vi "VersionCompareIn4Num.vi"(11 "VersionOnWeb":string) -> (3 "realFoundNew":bool)   [LabVIEW 2015]
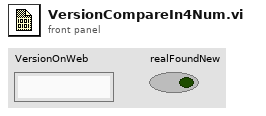
[diagram p1: front panel]
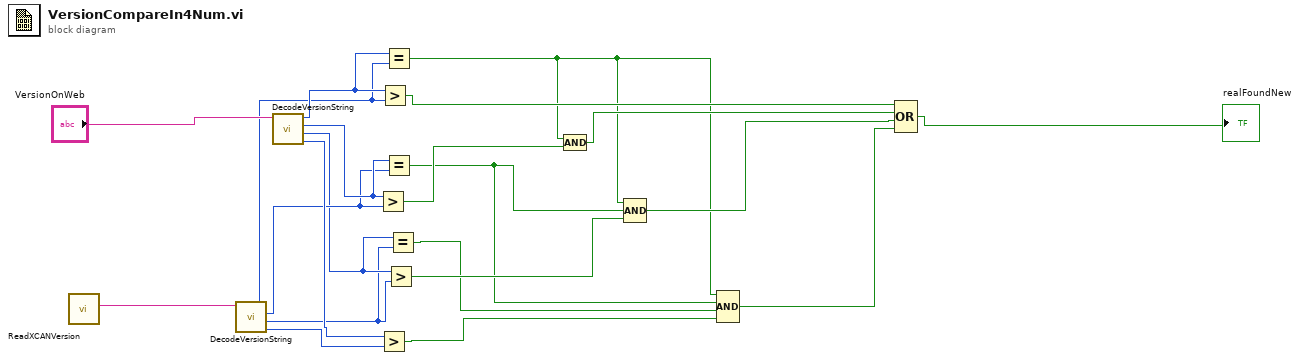
[diagram p0: block diagram]
diagram:
  n1 = call "ReadXCANVersion.vi"() -> ("Version"=w20:string)  [unwired: 9 in, 1 out]
  n2 = call "DecodeVersionString.vi"("VersionStr"=w20) -> ("build"=w18:i32, "correction"=w11:i32, "secondary"=w13:i32, "Main"=w15:i32)  [unwired: 5 in]
  n3 = call "DecodeVersionString.vi"("VersionStr"="VersionOnWeb") -> ("build"=w19:i32, "correction"=w12:i32, "secondary"=w14:i32, "Main"=w16:i32)  [unwired: 5 in]
  n4 = Greater?(x=w14, y=w13) -> (0:w9:bool)
  n5 = Greater?(x=w19, y=w18) -> (0:w2:bool)
  n6 = Greater?(x=w16, y=w15) -> (0:w17:bool)
  n7 = Equal?(x=w16, y=w15) -> (x = y?=w5:bool)
  n8 = Equal?(x=w14, y=w13) -> (x = y?=w4:bool)
  n9 = Greater?(x=w12, y=w11) -> (0:w7:bool)
  n10 = Equal?(x=w12, y=w11) -> (x = y?=w3:bool)
  n11 = Compound Arithmetic op=AND ("复合运算")(w5, w9) -> (w8:bool)
  n12 = Compound Arithmetic op=AND ("复合运算")(w5, w4, w7) -> (w6:bool)
  n13 = Compound Arithmetic op=AND ("复合运算")(w5, w4, w3, w2) -> (w1:bool)
  n14 = Compound Arithmetic op=OR ("复合运算")(w17, w8, w6, w1) -> (→"realFoundNew":bool)
